vi "Prep Acquisition.vi"(7 "Trigger Jitter (ms)":dbl, 8 "error in (no error)":errorcluster, 10 "Camera Settings":T1={"Exposure Time (ms)"=100.0, "Binning"=enum."2x2", "Scan Mode"=0, "Frames to Acquire"=1000.0, "Pixel Correction"=FALSE, "Frames to Skip"=0, "File Path"=path "", "Duty cycle"=0.0, "ALEX"=FALSE, "Shutter Enable"=[], "fluidics trigger frame"=0, "Bit Depth"=0, "Image Width (px)"=0, "Image Height (px)"=0, "Horizontal Offset (px)"=0, "Vertical Offset (px)"=0} {"fluidics trigger frame" max=60000 step=1; "Exposure Time (ms)" min=1.0 max=10000.0 step=1.0}, 11 "Camera in":refnum<class "Camera.lvclass">) -> (0 "error out":errorcluster, 3 "Camera out":refnum<class "Camera.lvclass">)   [LabVIEW 2023, in "Photometrics Camera.lvlib"]
uses:
  Photometrics Camera.lvlib
  Users/Public/Documents/Photometrics/TPM-LabVIEWSamples BETA/TPM LabVIEW adapter/Camera/Camera.lvclass
  Resources/Type Defs/Camera Settings.ctl
  Users/Public/Documents/Photometrics/TPM-LabVIEWSamples BETA/TPM LabVIEW adapter/SDK/Controls/All Params IDs.ctl
  Users/Public/Documents/Photometrics/TPM-LabVIEWSamples BETA/TPM LabVIEW adapter/SDK/Enum params values/ENUMS/ENUM EXP RES MODES.ctl
  Users/Public/Documents/Photometrics/TPM-LabVIEWSamples BETA/TPM LabVIEW adapter/SDK/Controls/Numeric Params IDs.ctl
  Users/Public/Documents/Photometrics/TPM-LabVIEWSamples BETA/TPM LabVIEW adapter/SDK/Enum params values/RINGS/RING EXPOSURE MODES.ctl
  Users/Public/Documents/Photometrics/TPM-LabVIEWSamples BETA/TPM LabVIEW adapter/SDK/Enum params values/ENUMS/ENUM EXPOSE OUT MODES.ctl
  Resources/GLOBAL/GLOBAL Experiment Metadata.vi
  Resources/GLOBAL/GLOBAL Time-critical.vi
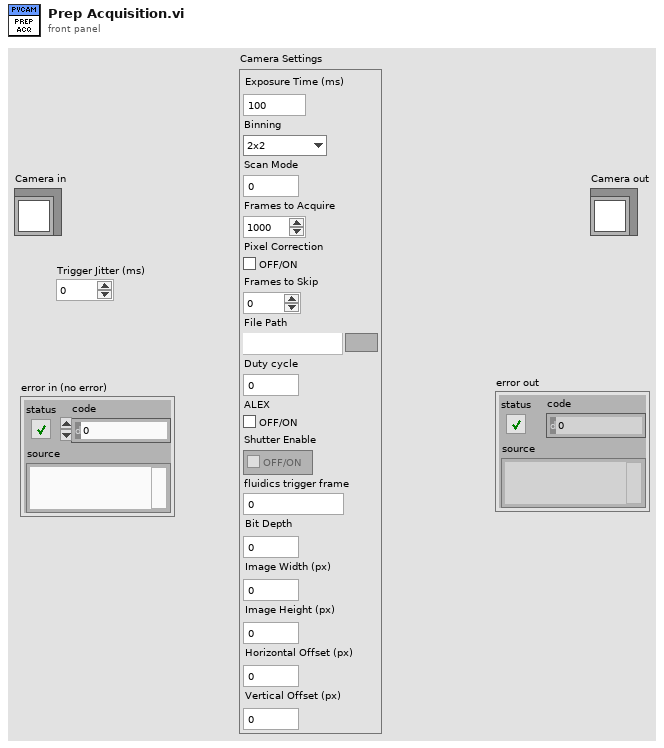
[diagram p1: front panel]
types:
  T1 = typedef "Camera Settings.ctl" = cluster{"Exposure Time (ms)":dbl, "Binning":enum16{"1x1", "2x2", "4x4"}, "Scan Mode":i32, "Frames to Acquire":dbl, "Pixel Correction":bool, "Frames to Skip":u32, "File Path":path, "Duty cycle":dbl, "ALEX":bool, "Shutter Enable":bool[], "fluidics trigger frame":u16, "Bit Depth":u16, "Image Width (px)":u16, "Image Height (px)":u16, "Horizontal Offset (px)":u16, "Vertical Offset (px)":u16}
  T2 = typedef "ENUM EXP RES MODES.ctl" = enum32{"EXP_RES_ONE_MILLISEC", "EXP_RES_ONE_MICROSEC", "EXP_RES_ONE_SEC"}
  T3 = enum32{"Sensitivity (12-bit)", "Speed (8-bit)", "Dynamic Range (16-bit)", "Sub-Electron (16-bit)"}
  T4 = typedef "ENUM EXPOSE OUT MODES.ctl" = enum32{"EXPOSE_OUT_FIRST_ROW", "EXPOSE_OUT_ALL_ROWS", "EXPOSE_OUT_ANY_ROW", "EXPOSE_OUT_ROLLING_SHUTTER", "EXPOSE_OUT_LINE_TRIGGER", "EXPOSE_OUT_GLOBAL_SHUTTER", "MAX_EXPOSE_OUT_MODE"}
  T5 = typedef "Numeric Params IDs.ctl" = i32
  T6 = typedef "All Params IDs.ctl" = i32
  T7 = typedef "RING EXPOSURE MODES.ctl" = u32
  T8 = typedef "Region.ctl" = cluster{"Origin X":u16, "Origin Y":u16, "Width":u16, "Height":u16}
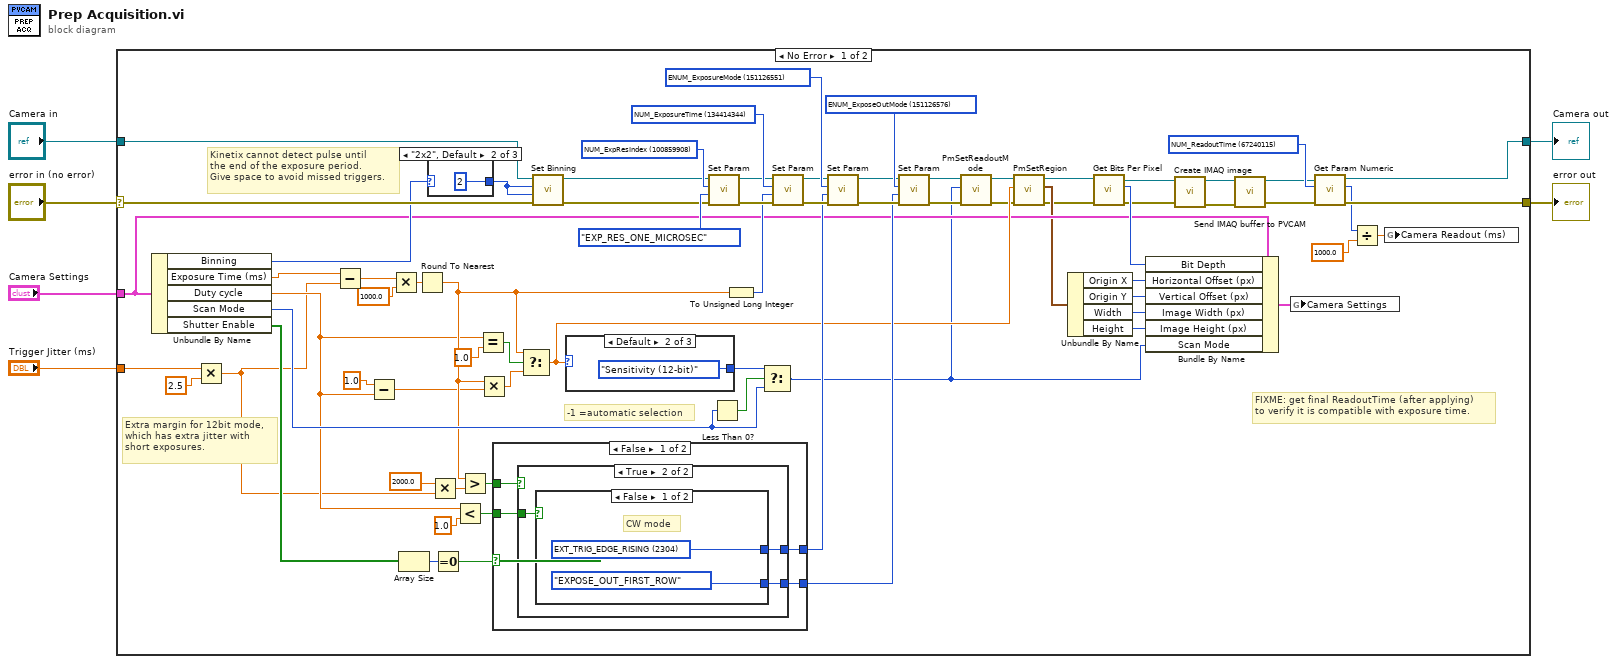
[diagram p0: block diagram]
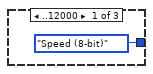
[diagram p2: hidden frame]
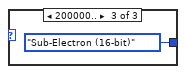
[diagram p3: hidden frame]
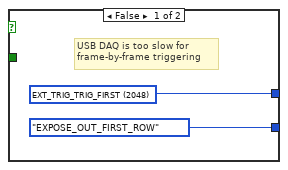
[diagram p4: hidden frame]
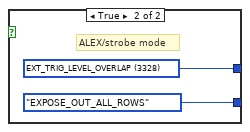
[diagram p5: hidden frame]
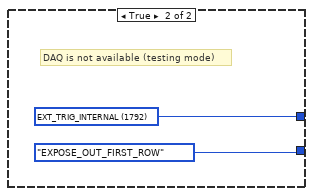
[diagram p6: hidden frame]
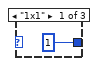
[diagram p7: hidden frame]
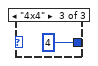
[diagram p8: hidden frame]
diagram:
  n1 = case shown="No Error" "error in (no error)" {
    selector: "error in (no error)" -> [w62 w102]
    tunnel: [w21 w102] -> w5
    tunnel: "Camera in" -> [w63 w101]
    tunnel: [w15 w101] -> w3
    tunnel: "Camera Settings" -> [w37 _]
    tunnel: "Trigger Jitter (ms)" -> [w9 _]
    frame No Error {
      w20 = T5 67240115 items=["NUM_ActualGain"=100794912, "NUM_AdcOffset"=16908483, "NUM_BitDepth"=16908799, "NUM_BofEofCount"=117637126, "NUM_CamFwVersion"=100794900, "NUM_CentroidsCount"=100860076, "NUM_CentroidsRadius"=100860075, "NUM_CentroidsThreshold"=117637295, "NUM_ClearCycles"=100794465, "NUM_ClearingTime"=268566708, "NUM_DdInfoLength"=16777217, "NUM_DdRetries"=100663299, "NUM_DdTimeout"=100663300, "NUM_DdVersion"=100663298, "NUM_ExpResIndex"=100859908, "NUM_ExposureTime"=134414344, "NUM_FrameBufferSize"=134414636, "NUM_FwellCapacity"=117572090, "NUM_GainIndex"=16908800, "NUM_GainMultFactor"=100794905, "NUM_IoAddr"=100794895, "NUM_IoBitDepth"=100794899, "NUM_IoState"=67240466, "NUM_LastMuxedSignal"=84082869, "NUM_ParSize"=100794425, "NUM_PciFwVersion"=100794902, "NUM_PixParDist"=100794868, "NUM_PixParSize"=100794431, "NUM_PixSerDist"=100794869, "NUM_PixSerSize"=100794430, "NUM_PixTime"=100794884, "NUM_PostTriggerDelay"=268566709, "NUM_Postmask"=100794422, "NUM_Postscan"=100794424, "NUM_PreTriggerDelay"=268566710, "NUM_PreampDelay"=100794870, "NUM_PreampOffControl"=117572091, "NUM_Premask"=100794421, "NUM_Prescan"=100794423, "NUM_ReadoutTime"=67240115, "NUM_RoiCount"=100860073, "NUM_SP_PpIndex"=16908831, "NUM_SP_PpParamIndex"=16908833, "NUM_ScanLineDelay"=100860157, "NUM_ScanLineTime"=268632318, "NUM_ScanWidth"=100860159, "NUM_SerSize"=100794426, "NUM_ShtrCloseDelay"=100794887, "NUM_ShtrOpenDelay"=100794888, "NUM_SmartStreamMode"=100795069, "NUM_SpdtabIndex"=16908801, "NUM_SummingWell"=184680953, "NUM_Temp"=16908813, "NUM_TempSetpoint"=16908814] ("Numeric Parameter")
      w72 = T6 100859908 items=["BOOL_BofEofClr"=184745991, "BOOL_CentroidsEnabled"=184746154, "BOOL_CircBuffer"=184746283, "BOOL_FrameCapable"=184680957, "BOOL_GainMultEnable"=184680989, "BOOL_MetadataEnabled"=184746152, "BOOL_MetadataResetTimestamp"=184746160, "BOOL_ScanDirectionReset"=184746236, "BOOL_SmartStreamModeEnabled"=184681148, "ENUM_BinningPar"=151191718, "ENUM_BinningSer"=151191717, "ENUM_BofEofEnable"=151191557, "ENUM_CamInterfaceMode"=150994955, "ENUM_CamInterfaceType"=150994954, "ENUM_CentroidsBgCount"=151191726, "ENUM_CentroidsMode"=151191725, "ENUM_ClearMode"=151126539, "ENUM_ColorMode"=151126520, "ENUM_CoolingMode"=151126230, "ENUM_ExpRes"=151191554, "ENUM_ExposeOutMode"=151126576, "ENUM_ExposureMode"=151126551, "ENUM_FanSpeedSetpoint"=151126726, "ENUM_FrameFlip"=151126273, "ENUM_FrameRotate"=151126272, "ENUM_ImageCompression"=151126265, "ENUM_ImageFormat"=151126264, "ENUM_IoDirection"=151126545, "ENUM_IoType"=151126544, "ENUM_MppCapable"=151126240, "ENUM_PMode"=151126540, "ENUM_ReadoutPort"=151126263, "ENUM_ScanDirection"=151191803, "ENUM_ScanMode"=151191802, "ENUM_ShtrOpenMode"=151126537, "ENUM_ShtrStatus"=151126538, "ENUM_TrigTabSignal"=151191732, "NUM_ActualGain"=100794912, "NUM_AdcOffset"=16908483, "NUM_BitDepth"=16908799, "NUM_BofEofCount"=117637126, "NUM_CamFwVersion"=100794900, "NUM_CentroidsCount"=100860076, "NUM_CentroidsRadius"=100860075, "NUM_CentroidsThreshold"=117637295, "NUM_ClearCycles"=100794465, "NUM_ClearingTime"=268566708, "NUM_DdInfoLength"=16777217, "NUM_DdRetries"=100663299, "NUM_DdTimeout"=100663300, "NUM_DdVersion"=100663298, "NUM_ExpResIndex"=100859908, "NUM_ExpTime"=100859905, "NUM_ExposureTime"=134414344, "NUM_FrameBufferSize"=134414636, "NUM_FwellCapacity"=117572090, "NUM_GainIndex"=16908800, "NUM_GainMultFactor"=100794905, "NUM_IoAddr"=100794895, "NUM_IoBitDepth"=100794899, "NUM_IoState"=67240466, "NUM_LastMuxedSignal"=84082869, "NUM_ParSize"=100794425, "NUM_PciFwVersion"=100794902, "NUM_PixParDist"=100794868, "NUM_PixParSize"=100794431, "NUM_PixSerDist"=100794869, "NUM_PixSerSize"=100794430, "NUM_PixTime"=100794884, "NUM_PostTriggerDelay"=268566709, "NUM_Postmask"=100794422, "NUM_Postscan"=100794424, "NUM_PreTriggerDelay"=268566710, "NUM_PreampDelay"=100794870, "NUM_PreampOffControl"=117572091, "NUM_Premask"=100794421, "NUM_Prescan"=100794423, "NUM_ReadoutTime"=67240115, "NUM_RoiCount"=100860073, "NUM_SP_PpIndex"=16908831, "NUM_SP_PpParamIndex"=16908833, "NUM_ScanLineDelay"=100860157, "NUM_ScanLineTime"=268632318, "NUM_ScanWidth"=100860159, "NUM_SerSize"=100794426, "NUM_ShtrCloseDelay"=100794887, "NUM_ShtrOpenDelay"=100794888, "NUM_SmartStreamMode"=100795069, "NUM_SpdtabIndex"=16908801, "NUM_SummingWell"=184680953, "NUM_Temp"=16908813, "NUM_TempSetpoint"=16908814, "PP_PpFeatId"=100794917, "PP_PpParam"=117572131, "PP_PpParamId"=100794918, "PP_ReadNoise"=100794916, "SS_SmartStreamDlyParams"=235012799, "SS_SmartStreamModeExpParams"=235012798, "STR_CamSystemsInfo"=218235416, "STR_CameraPartNumber"=218235013, "STR_ChipName"=218235009, "STR_DdInfo"=218103813, "STR_GainName"=218235394, "STR_HeadSerNumAlpha"=218235413, "STR_PpFeatName"=218235422, "STR_PpParamName"=218235426, "STR_ProductName"=218235012, "STR_SystemName"=218235010, "STR_VendorName"=218235011] ("PVCAM Param IDs")
      w77 = T6 151126576 items=["BOOL_BofEofClr"=184745991, "BOOL_CentroidsEnabled"=184746154, "BOOL_CircBuffer"=184746283, "BOOL_FrameCapable"=184680957, "BOOL_GainMultEnable"=184680989, "BOOL_MetadataEnabled"=184746152, "BOOL_MetadataResetTimestamp"=184746160, "BOOL_ScanDirectionReset"=184746236, "BOOL_SmartStreamModeEnabled"=184681148, "ENUM_BinningPar"=151191718, "ENUM_BinningSer"=151191717, "ENUM_BofEofEnable"=151191557, "ENUM_CamInterfaceMode"=150994955, "ENUM_CamInterfaceType"=150994954, "ENUM_CentroidsBgCount"=151191726, "ENUM_CentroidsMode"=151191725, "ENUM_ClearMode"=151126539, "ENUM_ColorMode"=151126520, "ENUM_CoolingMode"=151126230, "ENUM_ExpRes"=151191554, "ENUM_ExposeOutMode"=151126576, "ENUM_ExposureMode"=151126551, "ENUM_FanSpeedSetpoint"=151126726, "ENUM_FrameFlip"=151126273, "ENUM_FrameRotate"=151126272, "ENUM_ImageCompression"=151126265, "ENUM_ImageFormat"=151126264, "ENUM_IoDirection"=151126545, "ENUM_IoType"=151126544, "ENUM_MppCapable"=151126240, "ENUM_PMode"=151126540, "ENUM_ReadoutPort"=151126263, "ENUM_ScanDirection"=151191803, "ENUM_ScanMode"=151191802, "ENUM_ShtrOpenMode"=151126537, "ENUM_ShtrStatus"=151126538, "ENUM_TrigTabSignal"=151191732, "NUM_ActualGain"=100794912, "NUM_AdcOffset"=16908483, "NUM_BitDepth"=16908799, "NUM_BofEofCount"=117637126, "NUM_CamFwVersion"=100794900, "NUM_CentroidsCount"=100860076, "NUM_CentroidsRadius"=100860075, "NUM_CentroidsThreshold"=117637295, "NUM_ClearCycles"=100794465, "NUM_ClearingTime"=268566708, "NUM_DdInfoLength"=16777217, "NUM_DdRetries"=100663299, "NUM_DdTimeout"=100663300, "NUM_DdVersion"=100663298, "NUM_ExpResIndex"=100859908, "NUM_ExpTime"=100859905, "NUM_ExposureTime"=134414344, "NUM_FrameBufferSize"=134414636, "NUM_FwellCapacity"=117572090, "NUM_GainIndex"=16908800, "NUM_GainMultFactor"=100794905, "NUM_IoAddr"=100794895, "NUM_IoBitDepth"=100794899, "NUM_IoState"=67240466, "NUM_LastMuxedSignal"=84082869, "NUM_ParSize"=100794425, "NUM_PciFwVersion"=100794902, "NUM_PixParDist"=100794868, "NUM_PixParSize"=100794431, "NUM_PixSerDist"=100794869, "NUM_PixSerSize"=100794430, "NUM_PixTime"=100794884, "NUM_PostTriggerDelay"=268566709, "NUM_Postmask"=100794422, "NUM_Postscan"=100794424, "NUM_PreTriggerDelay"=268566710, "NUM_PreampDelay"=100794870, "NUM_PreampOffControl"=117572091, "NUM_Premask"=100794421, "NUM_Prescan"=100794423, "NUM_ReadoutTime"=67240115, "NUM_RoiCount"=100860073, "NUM_SP_PpIndex"=16908831, "NUM_SP_PpParamIndex"=16908833, "NUM_ScanLineDelay"=100860157, "NUM_ScanLineTime"=268632318, "NUM_ScanWidth"=100860159, "NUM_SerSize"=100794426, "NUM_ShtrCloseDelay"=100794887, "NUM_ShtrOpenDelay"=100794888, "NUM_SmartStreamMode"=100795069, "NUM_SpdtabIndex"=16908801, "NUM_SummingWell"=184680953, "NUM_Temp"=16908813, "NUM_TempSetpoint"=16908814, "PP_PpFeatId"=100794917, "PP_PpParam"=117572131, "PP_PpParamId"=100794918, "PP_ReadNoise"=100794916, "SS_SmartStreamDlyParams"=235012799, "SS_SmartStreamModeExpParams"=235012798, "STR_CamSystemsInfo"=218235416, "STR_CameraPartNumber"=218235013, "STR_ChipName"=218235009, "STR_DdInfo"=218103813, "STR_GainName"=218235394, "STR_HeadSerNumAlpha"=218235413, "STR_PpFeatName"=218235422, "STR_PpParamName"=218235426, "STR_ProductName"=218235012, "STR_SystemName"=218235010, "STR_VendorName"=218235011] ("PVCAM Param IDs")
      w78 = T6 151126551 items=["BOOL_BofEofClr"=184745991, "BOOL_CentroidsEnabled"=184746154, "BOOL_CircBuffer"=184746283, "BOOL_FrameCapable"=184680957, "BOOL_GainMultEnable"=184680989, "BOOL_MetadataEnabled"=184746152, "BOOL_MetadataResetTimestamp"=184746160, "BOOL_ScanDirectionReset"=184746236, "BOOL_SmartStreamModeEnabled"=184681148, "ENUM_BinningPar"=151191718, "ENUM_BinningSer"=151191717, "ENUM_BofEofEnable"=151191557, "ENUM_CamInterfaceMode"=150994955, "ENUM_CamInterfaceType"=150994954, "ENUM_CentroidsBgCount"=151191726, "ENUM_CentroidsMode"=151191725, "ENUM_ClearMode"=151126539, "ENUM_ColorMode"=151126520, "ENUM_CoolingMode"=151126230, "ENUM_ExpRes"=151191554, "ENUM_ExposeOutMode"=151126576, "ENUM_ExposureMode"=151126551, "ENUM_FanSpeedSetpoint"=151126726, "ENUM_FrameFlip"=151126273, "ENUM_FrameRotate"=151126272, "ENUM_ImageCompression"=151126265, "ENUM_ImageFormat"=151126264, "ENUM_IoDirection"=151126545, "ENUM_IoType"=151126544, "ENUM_MppCapable"=151126240, "ENUM_PMode"=151126540, "ENUM_ReadoutPort"=151126263, "ENUM_ScanDirection"=151191803, "ENUM_ScanMode"=151191802, "ENUM_ShtrOpenMode"=151126537, "ENUM_ShtrStatus"=151126538, "ENUM_TrigTabSignal"=151191732, "NUM_ActualGain"=100794912, "NUM_AdcOffset"=16908483, "NUM_BitDepth"=16908799, "NUM_BofEofCount"=117637126, "NUM_CamFwVersion"=100794900, "NUM_CentroidsCount"=100860076, "NUM_CentroidsRadius"=100860075, "NUM_CentroidsThreshold"=117637295, "NUM_ClearCycles"=100794465, "NUM_ClearingTime"=268566708, "NUM_DdInfoLength"=16777217, "NUM_DdRetries"=100663299, "NUM_DdTimeout"=100663300, "NUM_DdVersion"=100663298, "NUM_ExpResIndex"=100859908, "NUM_ExpTime"=100859905, "NUM_ExposureTime"=134414344, "NUM_FrameBufferSize"=134414636, "NUM_FwellCapacity"=117572090, "NUM_GainIndex"=16908800, "NUM_GainMultFactor"=100794905, "NUM_IoAddr"=100794895, "NUM_IoBitDepth"=100794899, "NUM_IoState"=67240466, "NUM_LastMuxedSignal"=84082869, "NUM_ParSize"=100794425, "NUM_PciFwVersion"=100794902, "NUM_PixParDist"=100794868, "NUM_PixParSize"=100794431, "NUM_PixSerDist"=100794869, "NUM_PixSerSize"=100794430, "NUM_PixTime"=100794884, "NUM_PostTriggerDelay"=268566709, "NUM_Postmask"=100794422, "NUM_Postscan"=100794424, "NUM_PreTriggerDelay"=268566710, "NUM_PreampDelay"=100794870, "NUM_PreampOffControl"=117572091, "NUM_Premask"=100794421, "NUM_Prescan"=100794423, "NUM_ReadoutTime"=67240115, "NUM_RoiCount"=100860073, "NUM_SP_PpIndex"=16908831, "NUM_SP_PpParamIndex"=16908833, "NUM_ScanLineDelay"=100860157, "NUM_ScanLineTime"=268632318, "NUM_ScanWidth"=100860159, "NUM_SerSize"=100794426, "NUM_ShtrCloseDelay"=100794887, "NUM_ShtrOpenDelay"=100794888, "NUM_SmartStreamMode"=100795069, "NUM_SpdtabIndex"=16908801, "NUM_SummingWell"=184680953, "NUM_Temp"=16908813, "NUM_TempSetpoint"=16908814, "PP_PpFeatId"=100794917, "PP_PpParam"=117572131, "PP_PpParamId"=100794918, "PP_ReadNoise"=100794916, "SS_SmartStreamDlyParams"=235012799, "SS_SmartStreamModeExpParams"=235012798, "STR_CamSystemsInfo"=218235416, "STR_CameraPartNumber"=218235013, "STR_ChipName"=218235009, "STR_DdInfo"=218103813, "STR_GainName"=218235394, "STR_HeadSerNumAlpha"=218235413, "STR_PpFeatName"=218235422, "STR_PpParamName"=218235426, "STR_ProductName"=218235012, "STR_SystemName"=218235010, "STR_VendorName"=218235011] ("PVCAM Param IDs")
      w79 = T6 134414344 items=["BOOL_BofEofClr"=184745991, "BOOL_CentroidsEnabled"=184746154, "BOOL_CircBuffer"=184746283, "BOOL_FrameCapable"=184680957, "BOOL_GainMultEnable"=184680989, "BOOL_MetadataEnabled"=184746152, "BOOL_MetadataResetTimestamp"=184746160, "BOOL_ScanDirectionReset"=184746236, "BOOL_SmartStreamModeEnabled"=184681148, "ENUM_BinningPar"=151191718, "ENUM_BinningSer"=151191717, "ENUM_BofEofEnable"=151191557, "ENUM_CamInterfaceMode"=150994955, "ENUM_CamInterfaceType"=150994954, "ENUM_CentroidsBgCount"=151191726, "ENUM_CentroidsMode"=151191725, "ENUM_ClearMode"=151126539, "ENUM_ColorMode"=151126520, "ENUM_CoolingMode"=151126230, "ENUM_ExpRes"=151191554, "ENUM_ExposeOutMode"=151126576, "ENUM_ExposureMode"=151126551, "ENUM_FanSpeedSetpoint"=151126726, "ENUM_FrameFlip"=151126273, "ENUM_FrameRotate"=151126272, "ENUM_ImageCompression"=151126265, "ENUM_ImageFormat"=151126264, "ENUM_IoDirection"=151126545, "ENUM_IoType"=151126544, "ENUM_MppCapable"=151126240, "ENUM_PMode"=151126540, "ENUM_ReadoutPort"=151126263, "ENUM_ScanDirection"=151191803, "ENUM_ScanMode"=151191802, "ENUM_ShtrOpenMode"=151126537, "ENUM_ShtrStatus"=151126538, "ENUM_TrigTabSignal"=151191732, "NUM_ActualGain"=100794912, "NUM_AdcOffset"=16908483, "NUM_BitDepth"=16908799, "NUM_BofEofCount"=117637126, "NUM_CamFwVersion"=100794900, "NUM_CentroidsCount"=100860076, "NUM_CentroidsRadius"=100860075, "NUM_CentroidsThreshold"=117637295, "NUM_ClearCycles"=100794465, "NUM_ClearingTime"=268566708, "NUM_DdInfoLength"=16777217, "NUM_DdRetries"=100663299, "NUM_DdTimeout"=100663300, "NUM_DdVersion"=100663298, "NUM_ExpResIndex"=100859908, "NUM_ExpTime"=100859905, "NUM_ExposureTime"=134414344, "NUM_FrameBufferSize"=134414636, "NUM_FwellCapacity"=117572090, "NUM_GainIndex"=16908800, "NUM_GainMultFactor"=100794905, "NUM_IoAddr"=100794895, "NUM_IoBitDepth"=100794899, "NUM_IoState"=67240466, "NUM_LastMuxedSignal"=84082869, "NUM_ParSize"=100794425, "NUM_PciFwVersion"=100794902, "NUM_PixParDist"=100794868, "NUM_PixParSize"=100794431, "NUM_PixSerDist"=100794869, "NUM_PixSerSize"=100794430, "NUM_PixTime"=100794884, "NUM_PostTriggerDelay"=268566709, "NUM_Postmask"=100794422, "NUM_Postscan"=100794424, "NUM_PreTriggerDelay"=268566710, "NUM_PreampDelay"=100794870, "NUM_PreampOffControl"=117572091, "NUM_Premask"=100794421, "NUM_Prescan"=100794423, "NUM_ReadoutTime"=67240115, "NUM_RoiCount"=100860073, "NUM_SP_PpIndex"=16908831, "NUM_SP_PpParamIndex"=16908833, "NUM_ScanLineDelay"=100860157, "NUM_ScanLineTime"=268632318, "NUM_ScanWidth"=100860159, "NUM_SerSize"=100794426, "NUM_ShtrCloseDelay"=100794887, "NUM_ShtrOpenDelay"=100794888, "NUM_SmartStreamMode"=100795069, "NUM_SpdtabIndex"=16908801, "NUM_SummingWell"=184680953, "NUM_Temp"=16908813, "NUM_TempSetpoint"=16908814, "PP_PpFeatId"=100794917, "PP_PpParam"=117572131, "PP_PpParamId"=100794918, "PP_ReadNoise"=100794916, "SS_SmartStreamDlyParams"=235012799, "SS_SmartStreamModeExpParams"=235012798, "STR_CamSystemsInfo"=218235416, "STR_CameraPartNumber"=218235013, "STR_ChipName"=218235009, "STR_DdInfo"=218103813, "STR_GainName"=218235394, "STR_HeadSerNumAlpha"=218235413, "STR_PpFeatName"=218235422, "STR_PpParamName"=218235426, "STR_ProductName"=218235012, "STR_SystemName"=218235010, "STR_VendorName"=218235011] ("PVCAM Param IDs")
      # "Extra margin for 12bit mode,\nwhich has extra jitter with\nshort exposures."
      # "Kinetix cannot detect pulse until\nthe end of the exposure period.\nGive space to avoid missed triggers."
      # "FIXME: get final ReadoutTime (after applying)\nto verify it is compatible with exposure time."
      # "-1 =automatic selection"
      n2 = Unbundle By Name(w37) -> ("Binning"=w58:enum16{"1x1", "2x2", "4x4"}, "Exposure Time (ms)"=w12:dbl, "Duty cycle"=w28:dbl, "Scan Mode"=w50:i32, "Shutter Enable"=w10:bool[])
      n3 = Multiply(x=w9, y=2.5) -> (x*y=w8:dbl)
      n4 = Subtract(x=w12, y=w8) -> (x-y=w11:dbl)
      n5 = Subtract(x=1.0, y=w28) -> (x-y=w27:dbl)
      n6 = Multiply(x=w11, y=1000.0) -> (x*y=w60:dbl)
      n7 = Array Size(array=w10) -> (size(s)=w61:i32)
      n8 = Round To Nearest(number=w60) -> (nearest integer value=w46:dbl)
      n9 = case shown="\"2x2\", Default" w58 {
        tunnel: [u16 1 ("Value in") u16 2 ("Value in") u16 4 ("Value in")] -> w44
        frame "1x1" {
        }
        frame "2x2", Default {
        }
        frame "4x4" {
        }
      }
      n10 = Multiply(x=2000.0 ("y"), y=w8) -> (x*y=w13:dbl)
      n11 = Equal To 0?(x=w61) -> (x = 0?=w54:bool)
      n12 = Less?(x=w28, y=1.0) -> (x < y?=w56:bool)
      n13 = Greater?(x=w46, y=w13) -> (0:w57:bool)
      n14 = Equal?(x=w28, y=1.0 ("x")) -> (x = y?=w53:bool)
      n15 = Multiply(x=w46, y=w27) -> (x*y=w29:dbl)
      n16 = case shown="False" w54 {
        tunnel: [w86 w96] -> w47
        tunnel: w56 -> [w85 _]
        tunnel: w57 -> [w84 _]
        tunnel: [w83 ENUM_EXPOSE_OUT_MODES."EXPOSE_OUT_FIRST_ROW" ("ENUM Expose Out Modes")] -> w48
        frame False {
          n17 = case shown="True" w84 {
            tunnel: [w87 w91] -> w86
            tunnel: w85 -> [_ w90]
            tunnel: [ENUM_EXPOSE_OUT_MODES."EXPOSE_OUT_FIRST_ROW" ("ENUM Expose Out Modes") w89] -> w83
            frame False {
              w87 = T7 2048 items=["TIMED_MODE"=0, "STROBED_MODE"=1, "BULB_MODE"=2, "TRIGGER_FIRST_MODE"=3, "FLASH_MODE"=4, "VARIABLE_TIMED_MODE"=5, "INT_STROBE_MODE"=6, "MAX_EXPOSE_MODE"=7, "EXT_TRIG_INTERNAL"=1792, "EXT_TRIG_TRIG_FIRST"=2048, "EXT_TRIG_EDGE_RISING"=2304, "EXT_TRIG_LEVEL"=2560, "EXT_TRIG_SOFTWARE_FIRST"=2816, "EXT_TRIG_SOFTWARE_EDGE"=3072, "EXT_TRIG_LEVEL_OVERLAP"=3328, "EXT_TRIG_LEVEL_PULSED"=3584] ("RING Exposure Modes")
              # "USB DAQ is too slow for \nframe-by-frame triggering"
            }
            frame True {
              n18 = case shown="False" w90 {
                tunnel: [w93 w95] -> w91
                tunnel: [ENUM_EXPOSE_OUT_MODES."EXPOSE_OUT_FIRST_ROW" ("ENUM Expose Out Modes") ENUM_EXPOSE_OUT_MODES."EXPOSE_OUT_ALL_ROWS" ("ENUM Expose Out Modes")] -> w89
                frame False {
                  w93 = T7 2304 items=["TIMED_MODE"=0, "STROBED_MODE"=1, "BULB_MODE"=2, "TRIGGER_FIRST_MODE"=3, "FLASH_MODE"=4, "VARIABLE_TIMED_MODE"=5, "INT_STROBE_MODE"=6, "MAX_EXPOSE_MODE"=7, "EXT_TRIG_INTERNAL"=1792, "EXT_TRIG_TRIG_FIRST"=2048, "EXT_TRIG_EDGE_RISING"=2304, "EXT_TRIG_LEVEL"=2560, "EXT_TRIG_SOFTWARE_FIRST"=2816, "EXT_TRIG_SOFTWARE_EDGE"=3072, "EXT_TRIG_LEVEL_OVERLAP"=3328, "EXT_TRIG_LEVEL_PULSED"=3584] ("RING Exposure Modes")
                  # "CW mode"
                }
                frame True {
                  w95 = T7 3328 items=["TIMED_MODE"=0, "STROBED_MODE"=1, "BULB_MODE"=2, "TRIGGER_FIRST_MODE"=3, "FLASH_MODE"=4, "VARIABLE_TIMED_MODE"=5, "INT_STROBE_MODE"=6, "MAX_EXPOSE_MODE"=7, "EXT_TRIG_INTERNAL"=1792, "EXT_TRIG_TRIG_FIRST"=2048, "EXT_TRIG_EDGE_RISING"=2304, "EXT_TRIG_LEVEL"=2560, "EXT_TRIG_SOFTWARE_FIRST"=2816, "EXT_TRIG_SOFTWARE_EDGE"=3072, "EXT_TRIG_LEVEL_OVERLAP"=3328, "EXT_TRIG_LEVEL_PULSED"=3584] ("RING Exposure Modes")
                  # "ALEX/strobe mode"
                }
              }
            }
          }
        }
        frame True {
          w96 = T7 1792 items=["TIMED_MODE"=0, "STROBED_MODE"=1, "BULB_MODE"=2, "TRIGGER_FIRST_MODE"=3, "FLASH_MODE"=4, "VARIABLE_TIMED_MODE"=5, "INT_STROBE_MODE"=6, "MAX_EXPOSE_MODE"=7, "EXT_TRIG_INTERNAL"=1792, "EXT_TRIG_TRIG_FIRST"=2048, "EXT_TRIG_EDGE_RISING"=2304, "EXT_TRIG_LEVEL"=2560, "EXT_TRIG_SOFTWARE_FIRST"=2816, "EXT_TRIG_SOFTWARE_EDGE"=3072, "EXT_TRIG_LEVEL_OVERLAP"=3328, "EXT_TRIG_LEVEL_PULSED"=3584] ("RING Exposure Modes")
          # "DAQ is not available (testing mode)"
        }
      }
      n19 = Select(t=w46, s=w53, f=w29) -> (s? t:f=w45:dbl)
      n20 = call "Set Binning.vi"("error in (no error)"=w62, "Binning Y"=w44, "Binning X"=w44, "Camera in"=w63) -> ("error out"=w70:errorcluster, "Camera out"=w67:refnum<class "Camera.lvclass">)  [unwired: 6 in]
      n21 = case shown="Default" w45 {
        tunnel: [T3."Speed (8-bit)" ("Trigger Setting") T3."Sensitivity (12-bit)" ("Trigger Setting") T3."Sub-Electron (16-bit)" ("Trigger Setting")] -> w49
        frame ..12000 {
        }
        frame Default {
        }
        frame 200000.. {
        }
      }
      n22 = call "Set Param.vi"("error in (no error)"=w70, "Parameter value"=ENUM_EXP_RES_MODES."EXP_RES_ONE_MICROSEC" ("ENUM Exp Res Modes"), "PVCAM Param IDs"=w72, "Camera In"=w67) -> ("error out"=w69:errorcluster, "Camera Out"=w68:refnum<class "Camera.lvclass">)  [unwired: 6 in]
      n23 = Less Than 0?(x=w50) -> (x < 0?=w51:bool)
      n24 = To Unsigned Long Integer(number=w46) -> (unsigned 32bit integer=w66:u32)
      n25 = Select(t=w49, s=w51, f=w50) -> (s? t:f=w25:u32)
      n26 = call "Set Param.vi"("error in (no error)"=w69, "Parameter value"=w66, "PVCAM Param IDs"=w79, "Camera In"=w68) -> ("error out"=w73:errorcluster, "Camera Out"=w74:refnum<class "Camera.lvclass">)  [unwired: 6 in]
      n27 = call "Set Param.vi"("error in (no error)"=w73, "Parameter value"=w47, "PVCAM Param IDs"=w78, "Camera In"=w74) -> ("error out"=w76:errorcluster, "Camera Out"=w75:refnum<class "Camera.lvclass">)  [unwired: 6 in]
      n28 = call "Set Param.vi"("error in (no error)"=w76, "Parameter value"=w48, "PVCAM Param IDs"=w77, "Camera In"=w75) -> ("error out"=w64:errorcluster, "Camera Out"=w65:refnum<class "Camera.lvclass">)  [unwired: 6 in]
      n29 = call "PmSetReadoutMode.vi"("error in (no error)"=w64, "Readout Mode"=w25, "Camera in"=w65) -> ("error out"=w23:errorcluster, "Camera out"=w24:refnum<class "Camera.lvclass">)  [unwired: 7 in]
      n30 = call "PmSetRegion.vi"("error in (no error)"=w23, "Frame Time (us)"=w45, "Camera in"=w24) -> ("error out"=w32:errorcluster, "Region"=w36:T8, "Camera out"=w33:refnum<class "Camera.lvclass">)  [unwired: 6 in]
      n31 = Unbundle By Name(w36) -> ("Origin X"=w43:u16, "Origin Y"=w42:u16, "Width"=w41:u16, "Height"=w40:u16)
      n32 = call "Get Bits Per Pixel.vi"("error in (no error)"=w32, "Camera in"=w33) -> ("error out"=w30:errorcluster, "Bits Per Pixel"=w38:u32, "Camera out"=w31:refnum<class "Camera.lvclass">)  [unwired: 7 in]
      n33 = Bundle By Name(cluster=w37, "Bit Depth"=w38, "Horizontal Offset (px)"=w43, "Vertical Offset (px)"=w42, "Image Width (px)"=w41, "Image Height (px)"=w40, "Scan Mode"=w25) -> (w39:T1)
      n34 = call "Create IMAQ image.vi"("error in (no error)"=w30, "Camera in"=w31) -> ("error out"=w34:errorcluster, "Camera out"=w35:refnum<class "Camera.lvclass">)  [unwired: 8 in]
      n35 = call "Send IMAQ buffer to PVCAM.vi"("error in (no error)"=w34, "Camera in"=w35) -> ("error out"=w22:errorcluster, "Camera out"=w16:refnum<class "Camera.lvclass">)  [unwired: 8 in]
      n36 = global write "GLOBAL Experiment Metadata.vi" "Camera Settings"(w39) -> ()
      n37 = call "Get Param Numeric.vi"("error in (no error)"=w22, "Numeric Parameter"=w20, "Camera In"=w16) -> ("error out"=w21:errorcluster, "Value"=w18:i64, "Camera Out"=w15:refnum<class "Camera.lvclass">)  [unwired: 4 in, 2 out]
      n38 = Divide(x=w18, y=1000.0) -> (x/y=w19:dbl)
      n39 = global write "GLOBAL Time-critical.vi" "Camera Readout (ms)"(w19) -> ()
    }
    frame Error {
    }
  }
  "error out" <- w5
  "Camera out" <- w3
